vi "loadcell data read.vi"(8 "error in (no error)":errorcluster, 11 "Refnum in":refnum<k21>) -> (0 "error out":errorcluster, 2 "Filtered x":dbl, 3 "Refnum out":refnum<k21>)   [LabVIEW 2021]
uses:
  <vilib>/Analysis/3filter.llb/Filter Passband Type.ctl
  <vilib>/DAQmx/read.llb/DAQmx Read (Analog DBL 1Chan 1Samp).vi
  <vilib>/DAQmx/miscellaneous.llb/DAQmx Fill In Error Info.vi
  <vilib>/ptbypt/NI_PtbyPt.lvlib
  <vilib>/Analysis/NI_AALBase.lvlib
panel:
  out "Numeric":dbl
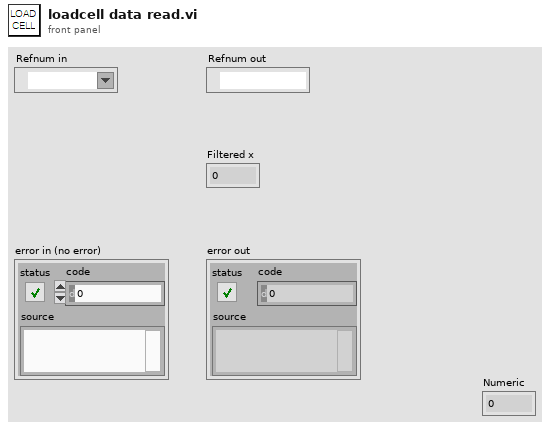
[diagram p1: front panel]
types:
  T1 = typedef "NI_AALBase.lvlib/Filter Passband Type.ctl" = enum32{"Lowpass", "Highpass", "Bandpass", "Bandstop"}
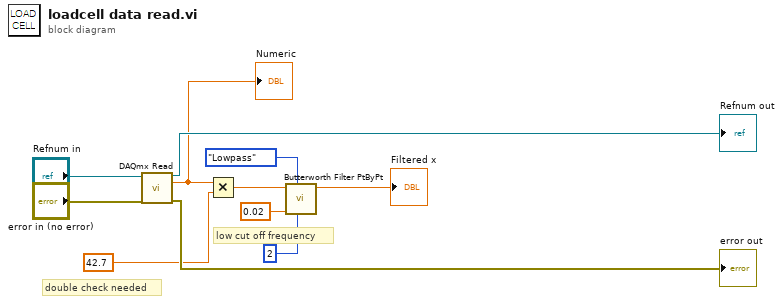
[diagram p0: block diagram]
diagram:
  # "double check needed"
  # "low cut off frequency"
  n1 = call-poly <vilib>:"DAQmx Read.vi"("task/channels in"="Refnum in", "error in"="error in (no error)") -> ("task out"=→"Refnum out":refnum<k21>, "data"=w1:dbl, "error out"=→"error out":errorcluster)  [unwired: 11 in]
  "Numeric" <- w1
  n2 = Multiply(x=w1, y=42.7) -> (x*y=w11:dbl)
  n3 = call <vilib>:"Butterworth Filter PtByPt.vi"("order"=2, "filter type"=Filter_Passband_Type."Lowpass", "low cutoff freq: fl"=0.02, "x"=w11) -> ("Filtered x"=→"Filtered x":dbl)  [unwired: 5 in, 1 out]
